vi "__goldopt_part2.vi"(9 "f2>f1":bool, 10 "f_changed":dbl, 11 "f_notchange":dbl) -> (2 "f2":dbl, 3 "f1":dbl)   [LabVIEW 2017]
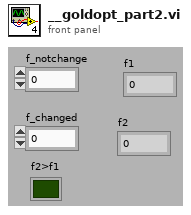
[diagram p1: front panel]
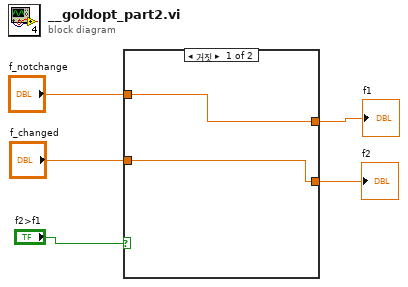
[diagram p0: block diagram]
diagram:
  n1 = case shown="거짓" "f2>f1" {
    tunnel: [w7 w9] -> w4
    tunnel: "f_notchange" -> [w6 w9]
    tunnel: [w6 w8] -> w2
    tunnel: "f_changed" -> [w7 w8]
    frame False {
    }
    frame True {
    }
  }
  "f1" <- w2
  "f2" <- w4
